vi "main.vi"() -> ()   [LabVIEW 2015, in "lv-launcher-nre.lvlib"]
uses:
  lv-launcher-nre.lvlib
  _controls/event.ctl
  _controls/event_command.ctl
panel:
  out "error":errorcluster
  # "<<Splash Screen>>"
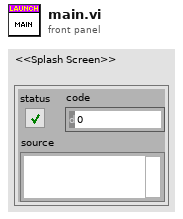
[diagram p1: front panel]
types:
  T1 = typedef "lv-launcher-nre.lvlib/event_command.ctl" = enum16{"<command>", "die", "<null>"}
  T2 = typedef "lv-launcher-nre.lvlib/event.ctl" = cluster{"command":T1, "data":variant}
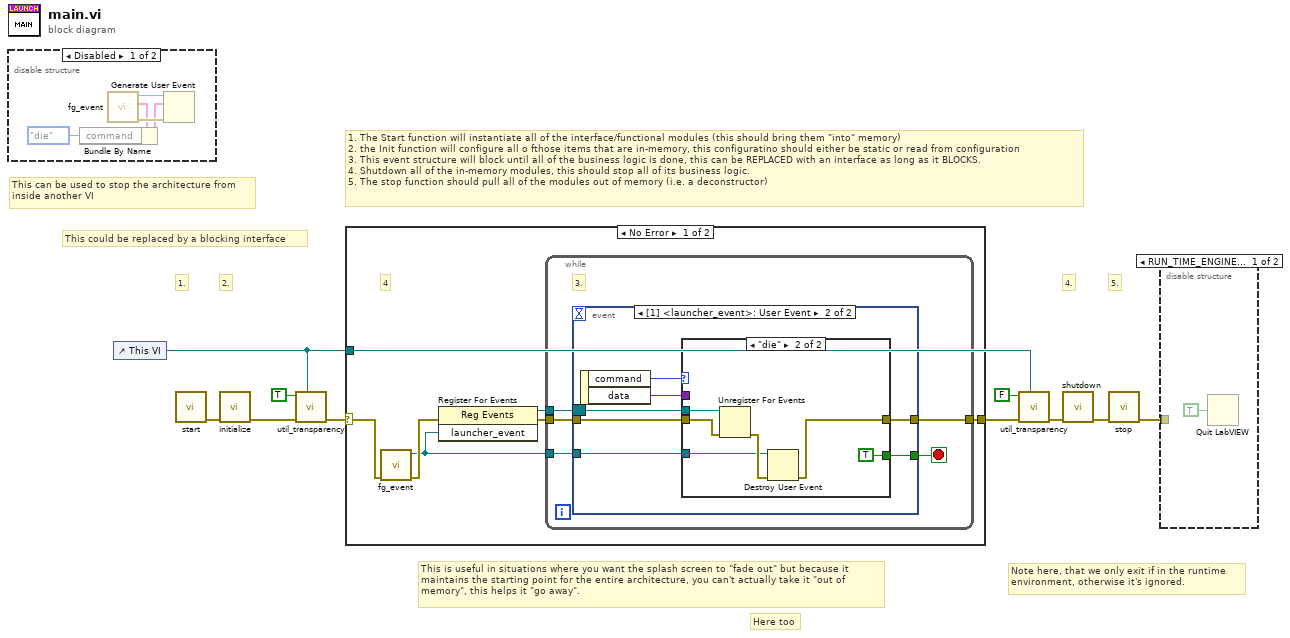
[diagram p0: block diagram]
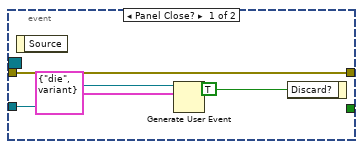
[diagram p3: hidden frame]
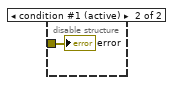
[diagram p6: hidden frame]
diagram:
  # "This can be used to stop the architecture from\ninside another VI"
  # "Note here, that we only exit if in the runtime\nenvironment, otherwise it's ignored."
  # "This could be replaced by a blocking interface"
  # "1. The Start function will instantiate all of the interface/functional modules (this should bring them \"into\" memory)\n2. the Init function will configure all o fthose items that are in-memory, this configuratino should either be static or read from configuration\n3. This event structure will block until all of the business logic is done, this can be REPLACED with an interface as long as it BLOCKS.\n4. Shutdown all of the in-memory modules, this should stop all of its business logic.\n5. The stop function should pull all of the modules out of memory (i.e. a deconstructor)"
  # "5."
  # "4."
  # "Here too"
  # "This is useful in situations where you want the splash screen to \"fade out\" but because it\nmaintains the starting point for the entire architecture, you can't actually take it \"out of \nmemory\", this helps it \"go away\"."
  # "2."
  # "1."
  n1 = disable-structure shown="Disabled" {
    frame Disabled {
      n2 = call "fg_event.vi"() -> ("error out"=w15:errorcluster, "data"=w13:T2, "launcher_event"=w14:refnum<user-event>)  [unwired: 9 in]
      n3 = Bundle By Name(cluster=w13, "command"=event_command."die" ("Command")) -> (w12:T2)
      n4 = Generate User Event(user event=w14, event data cluster=w12, error in=w15) -> ()  [unwired: 1 in, 2 out]
    }
    frame Enabled {
    }
  }
  n5 = control-ref of="This VI"() -> (w5:refnum<vi>)
  n6 = call "start.vi"() -> ("error out"=w10:errorcluster)  [unwired: 11 in]
  n7 = call "initialize.vi"("error in (no error)"=w10) -> ("error out"=w4:errorcluster)  [unwired: 10 in]
  n8 = call "util_transparency.vi"("vi_reference"=w5, "error in (no error)"=w4, "opaque_transparent"=TRUE) -> ("error out"=w1:errorcluster)  [unwired: 8 in]
  n9 = case shown="No Error" w1 {
    selector: w1 -> [w17 w45]
    tunnel: [w20 w45] -> w6
    tunnel: w5 -> [_ _]
    frame No Error {
      # "4"
      n10 = call "fg_event.vi"("error in (no error)"=w17) -> ("error out"=w21:errorcluster, "launcher_event"=w16:refnum<user-event>)  [unwired: 8 in, 1 out]
      n11 = register-events(error in=w21, w16) -> (reference out=w19:refnum<event-registration>, error out=w18:errorcluster)  [unwired: 1 in]
      n12 = while {
        tunnel: w19 -> [w24]
        tunnel: w18 -> [w26]
        tunnel: [w25] -> w20
        tunnel: w16 -> [w22]
        stop <- w23 stop-if-true
        # "3."
        n13 = event shown="[1] <launcher_event>: User Event" {
          selector: w24 -> [_ w32]
          dyn-events: _ -> [_ _]
          timeout: _ -> [_ _]
          tunnel: w26 -> [w30 w34]
          tunnel: [w30 w35] -> w25
          tunnel: [_ w36] -> w23
          tunnel: w22 -> [w28 w31]
          event Panel Close? {
            n14 = event-data() -> ()  [unwired: 1 in, 1 out]
            n15 = Generate User Event(user event=w28, event data cluster=T2 {"command"=enum."die", "data"=variant} ("event data")) -> ()  [unwired: 2 in, 2 out]
            n16 = event-data("Discard?"=TRUE) -> ()  [unwired: 1 in, 1 out]
          }
          event User Event {
            n17 = event-data() -> ("command"=w37:T1, "data"=w33:variant)  [unwired: 1 in]
            n18 = case shown="\"die\"" w37 {
              tunnel: [_ TRUE] -> w36
              tunnel: w34 -> [w38 w40]
              tunnel: [w38 w39] -> w35
              tunnel: w33 -> [_ _]
              tunnel: w32 -> [_ w41]
              tunnel: w31 -> [_ w42]
              frame Default {
              }
              frame "die" {
                n19 = Unregister For Events(event registration refnum=w41, error in=w40) -> (error out=w44:errorcluster)
                n20 = Destroy User Event(user event=w42, error in=w44) -> (error out=w39:errorcluster)
              }
            }
          }
        }
      }
    }
    frame Error {
    }
  }
  n21 = call "util_transparency.vi"("vi_reference"=w5, "error in (no error)"=w6, "opaque_transparent"=FALSE) -> ("error out"=w7:errorcluster)  [unwired: 8 in]
  n22 = call "shutdown.vi"("error in (no error)"=w7) -> ("error out"=w8:errorcluster)  [unwired: 10 in]
  n23 = call "stop.vi"("error in (no error)"=w8) -> ("error out"=w9:errorcluster)  [unwired: 10 in]
  n24 = disable-structure shown="RUN_TIME_ENGINE==True" {
    disable-tunnel: w9 -> [_ w47]
    frame condition #0 {
      n25 = Quit LabVIEW(quit? (T)=TRUE) -> ()
    }
    frame condition #1 (active) {
      "error" <- w47
    }
  }
